vi "Example.vi"() -> ()   [LabVIEW 2015, in "rtlsdr.lvlib"]
uses:
  rtlsdr.lvlib
  <vilib>/measure/NI_MAPro.lvlib
  <vilib>/Analysis/4window.llb/windowTd.ctl
  <vilib>/Analysis/NI_AALPro.lvlib
  <vilib>/measure/maspectr.llb/FFT Power Spectrum and PSD for 1 Chan (CDB).vi
panel:
  out "Waveform Graph":cluster{"f0":dbl, "df":dbl, "magnitude":dbl[]}(graph)
  in  "stop":bool
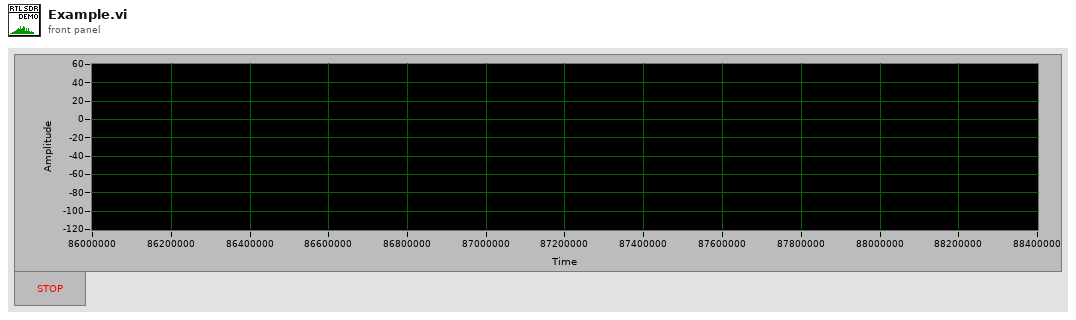
[diagram p1: front panel]
types:
  T1 = typedef "NI_AALPro.lvlib/windowTd.ctl" = u32
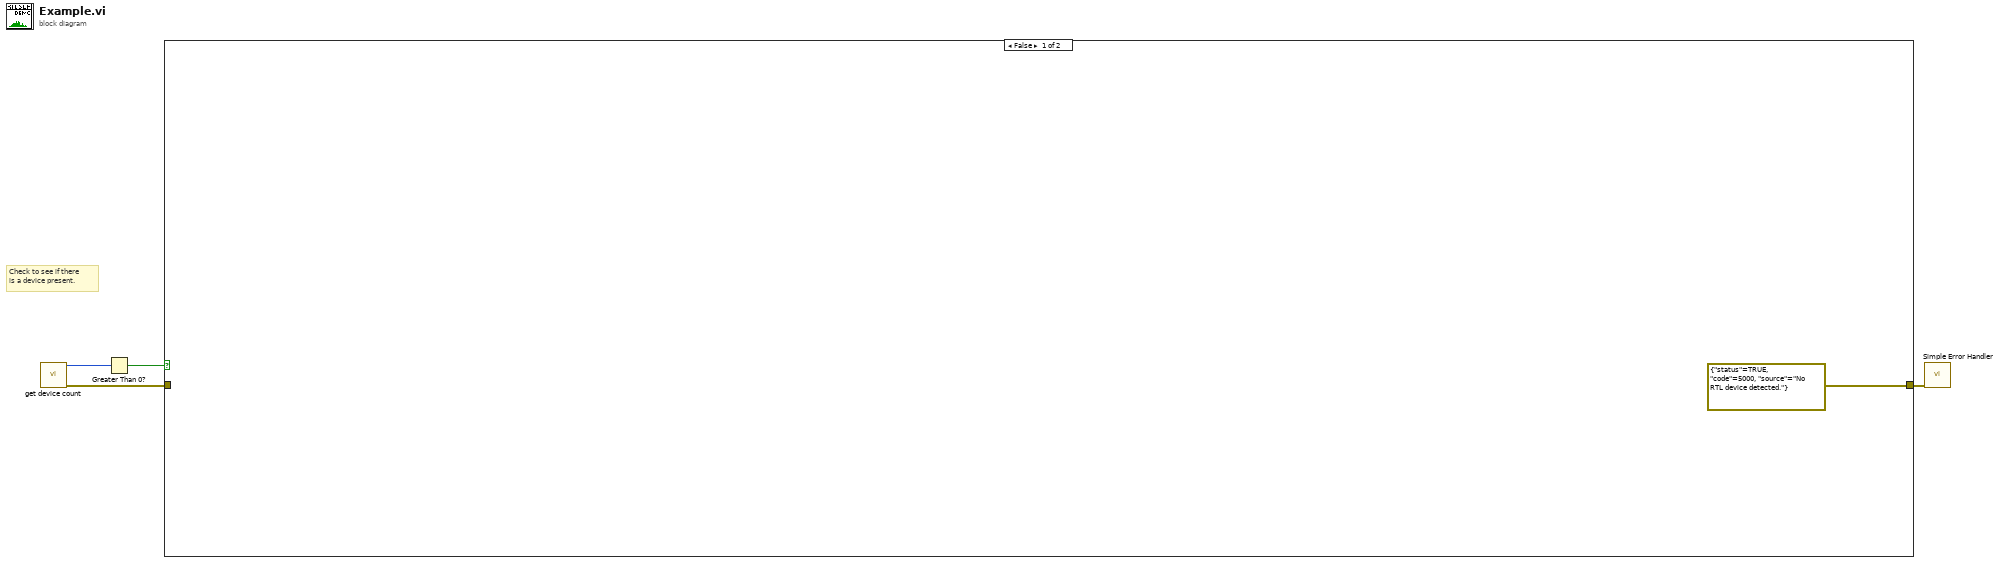
[diagram p0: block diagram]
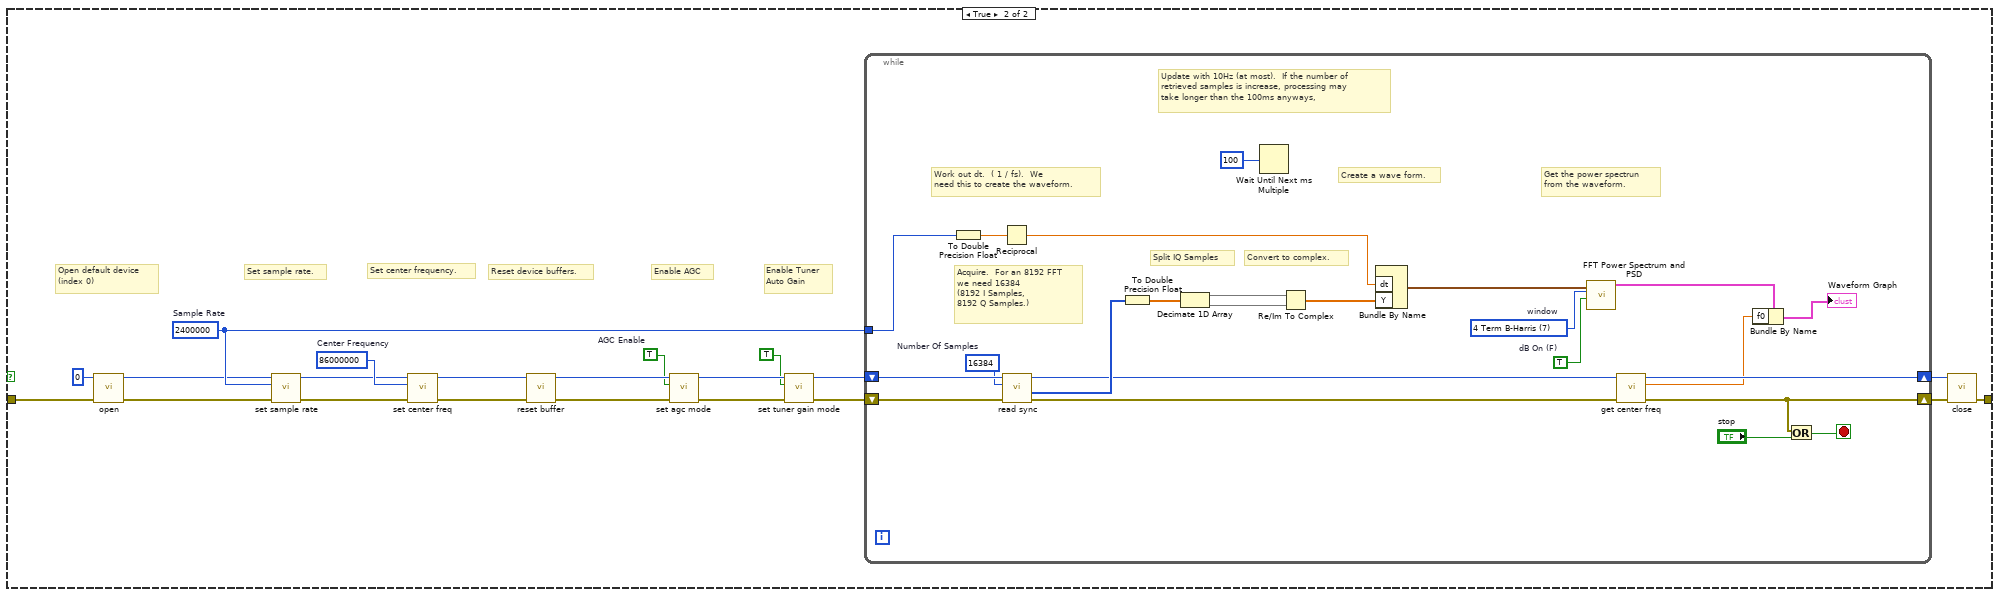
[diagram p2: hidden frame]
diagram:
  # "Check to see if there\nis a device present."
  n1 = call "get device count.vi"() -> ("error out"=w3:errorcluster, "Device Count"=w2:u32)  [unwired: 10 in]
  n2 = Greater Than 0?(x=w2) -> (x > 0?=w1:bool)
  n3 = case shown="False" w1 {
    tunnel: [errorcluster {"status"=TRUE, "code"=5000, "source"="No RTL device detected."} ("error out") w9] -> w4
    tunnel: w3 -> [_ w8]
    frame False {
    }
    frame True {
      w12 = u32 86000000  # Center Frequency
      w18 = TRUE  # AGC Enable
      w23 = u32 2400000  # Sample Rate
      # "Enable Tuner\nAuto Gain"
      # "Enable AGC"
      # "Reset device buffers."
      # "Set center frequency."
      # "Set sample rate."
      # "Open default device\n(index 0)"
      n4 = call "open.vi"("error in (no error)"=w8, "Device Index"=u32 0 ("index")) -> ("error out"=w13:errorcluster, "DeviceRefnum Out"=w14:u64)  [unwired: 6 in]
      n5 = call "set sample rate.vi"("error in (no error)"=w13, "Sample Rate"=w23, "DeviceRefnum"=w14) -> ("error out"=w11:errorcluster, "DeviceRefnum Out"=w10:u64)  [unwired: 6 in, 1 out]
      n6 = call "set center freq.vi"("error in (no error)"=w11, "Center Frequency"=w12, "DeviceRefnum"=w10) -> ("error out"=w16:errorcluster, "DeviceRefnum Out"=w15:u64)  [unwired: 6 in, 1 out]
      n7 = call "reset buffer.vi"("error in (no error)"=w16, "DeviceRefnum"=w15) -> ("error out"=w22:errorcluster, "DeviceRefnum Out"=w20:u64)  [unwired: 7 in, 1 out]
      n8 = call "set agc mode.vi"("error in (no error)"=w22, "AGC Enable"=w18, "DeviceRefnum"=w20) -> ("error out"=w21:errorcluster, "DeviceRefnum Out"=w19:u64)  [unwired: 6 in, 1 out]
      n9 = call "set tuner gain mode.vi"("error in (no error)"=w21, "AutoGain"=TRUE, "DeviceRefnum"=w19) -> ("error out"=w6:errorcluster, "DeviceRefnum Out"=w7:u64)  [unwired: 6 in, 1 out]
      n10 = while {
        tunnel: w23 -> [w40]
        shift-right: [w30] -> w24
        shift-left: w7 -> [w50]
        shift-right: [w29] -> w25
        shift-left: w6 -> [w49]
        stop <- w34 stop-if-true
        w39 = 16384  # Number Of Samples
        w42 = TRUE  # dB On (F)
        w43 = T1 7 items=["Rectangle"=0, "Hanning"=1, "Hamming"=2, "Blackman-Harris"=3, "Exact Blackman"=4, "Blackman"=5, "Flat Top"=6, "4 Term B-Harris "=7, "7 Term B-Harris"=8, "Low Sidelobe"=9, "Blackman Nuttall"=11, "Triangle"=30, "Bartlett-Hanning"=31, "Bohman"=32, "Parzen"=33, "Welch"=34, "Kaiser"=60, "Dolph-Chebyshev"=61, "Gaussian"=62]  # window
        # "Update with 10Hz (at most).  If the number of \nretrieved samples is increase, processing may\ntake longer than the 100ms anyways,"
        # "Get the power spectrun\nfrom the waveform."
        # "Acquire.  For an 8192 FFT\nwe need 16384 \n(8192 I Samples,\n8192 Q Samples.)"
        # "Create a wave form."
        # "Convert to complex."
        # "Split IQ Samples"
        # "Work out dt.  ( 1 / fs).  We\nneed this to create the waveform."
        n11 = To Double Precision Float(number=w40) -> (double precision float=w44:dbl)
        n12 = Reciprocal(x=w44) -> (1/x=w37:dbl)
        n13 = call "read sync.vi"("error in (no error)"=w49, "Number Of Samples"=w39, "DeviceRefnum"=w50) -> ("error out"=w32:errorcluster, "Sample Buffer"=w47:u8[], "DeviceRefnum Out"=w31:u64)  [unwired: 5 in, 1 out]
        n14 = To Double Precision Float(number=w47) -> (double precision float=w48:dbl[])
        n15 = Decimate 1D Array(w48) -> (w46:dbl[], w45:dbl[])
        n16 = Wait Until Next ms Multiple(millisecond multiple=u32 100) -> ()  [unwired: 1 out]
        n17 = Re/Im To Complex(1:w45, 2:w46) -> (0:w38:cdb[])
        n18 = Bundle By Name("dt"=w37, "Y"=w38) -> (w41:waveform(cdb))  [unwired: 1 in]
        n19 = call-poly <vilib>:"FFT Power Spectrum and PSD.vi"("dB On (F)"=w42, "window"=w43, "time signal"=w41) -> ("Power Spectrum / PSD"=w28:cluster{"f0":dbl, "df":dbl, "magnitude":dbl[]})  [unwired: 5 in, 3 out]
        n20 = call "get center freq.vi"("error in (no error)"=w32, "DeviceRefnum"=w31) -> ("error out"=w29:errorcluster, "Center Frequency"=w27:dbl, "DeviceRefnum Out"=w30:u64)  [unwired: 7 in]
        n21 = Bundle By Name(cluster=w28, "f0"=w27) -> (→"Waveform Graph":cluster{"f0":dbl, "df":dbl, "magnitude":dbl[]})
        n22 = Or(x=w29, y="stop") -> (x .or. y?=w34:bool)
      }
      n23 = call "close.vi"("error in (no error)"=w25, "DeviceRefnum"=w24) -> ("error out"=w9:errorcluster)  [unwired: 8 in, 1 out]
    }
  }
  n24 = call <vilib>:"Simple Error Handler.vi"("error in (no error)"=w4) -> ()  [unwired: 4 in, 5 out]
